vi "Global - Disable Hardware API Constant.vi"() -> ()   [LabVIEW 2020, in "AIM MIL-STD-1553 Hardware API.lvlib"]
uses:
  AIM MIL-STD-1553 Hardware API.lvlib
panel:
  out "Disable Hardware API":T1(ring)
  # "This should be kept Enabled\nCan be used by Unit Tests\nto skip HW API calls"
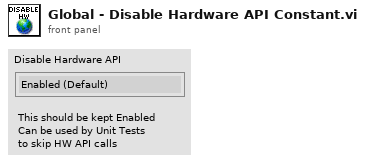
[diagram p1: front panel]
types:
  T1 = enum16{"Enabled (Default)", "Disabled for Unit Testing"}
diagram:
